vi "WILT Stave Status.vi"(0 "GUI Aisle 4":T3[](array[typedef]) {"Night Cycle Count" format="%04d"; "Day Cycle Count" format="%04d"}, 1 "Operation Type":enum16{"Write", "Read"}(ring), 2 "File Locations":T1[](array[typedef]), 5 "GUI Aisle 3":T3[](array[typedef]) {"Night Cycle Count" format="%04d"; "Day Cycle Count" format="%04d"}, 7 "GUI Aisle 2":T3[](array[typedef]) {"Night Cycle Count" format="%04d"; "Day Cycle Count" format="%04d"}, 9 "GUI Aisle 1 (SLAT)":T3[](array[typedef]) {"Night Cycle Count" format="%04d"; "Day Cycle Count" format="%04d"}, 11 "Error In":errorcluster, 12 "GUI Aisle 1A (SLAT)":T3[](array[typedef]) {"Night Cycle Count" format="%04d"; "Day Cycle Count" format="%04d"}) -> (4 "GUI Aisle 4 Out":T3[](array[typedef]) {"Night Cycle Count" format="%04d"; "Day Cycle Count" format="%04d"}, 6 "GUI Aisle 3 Out":T3[](array[typedef]) {"Night Cycle Count" format="%04d"; "Day Cycle Count" format="%04d"}, 8 "GUI Aisle 2 Out":T3[](array[typedef]) {"Night Cycle Count" format="%04d"; "Day Cycle Count" format="%04d"}, 10 "GUI Aisle 1 (SLAT) Out":T3[](array[typedef]) {"Night Cycle Count" format="%04d"; "Day Cycle Count" format="%04d"}, 14 "GUI Aisle 1A (SLAT) Out":T3[](array[typedef]) {"Night Cycle Count" format="%04d"; "Day Cycle Count" format="%04d"}, 15 "Error Out":errorcluster)   [LabVIEW 2016]
uses:
  Type Definitions/WILT Dryer.ctl
  Type Definitions/WILT Dryer Details.ctl
  Type Definitions/WILT Agilent Channel Definition.ctl
  Type Definitions/WILT DAQ Data.ctl
  Utility/Save File/File Setup (Public)/Type Definition/Save File DOE File Path Control.ctl
  Utility/Save File/File Setup (Public)/Type Definition/Save File DOE Data Save Filepaths.ctl
  <vilib>/Utility/file.llb/Write Delimited Spreadsheet (string).vi
  <vilib>/Utility/file.llb/Read Delimited Spreadsheet (string).vi
  Utility/Save File/File Setup.lvlib
panel:
  out "Info Table":string[][](array[string])
  # "Day"
  # "Night"
  # "Day"
  # "Night"
  # "Day"
  # "Night"
  # "Day"
  # "Night"
  # "Day"
  # "Night"
  # "Day"
  # "Night"
  # "Day"
  # "Night"
  # "Day"
  # "Night"
  # "Day"
  # "Night"
  # "Day"
  # "Night"
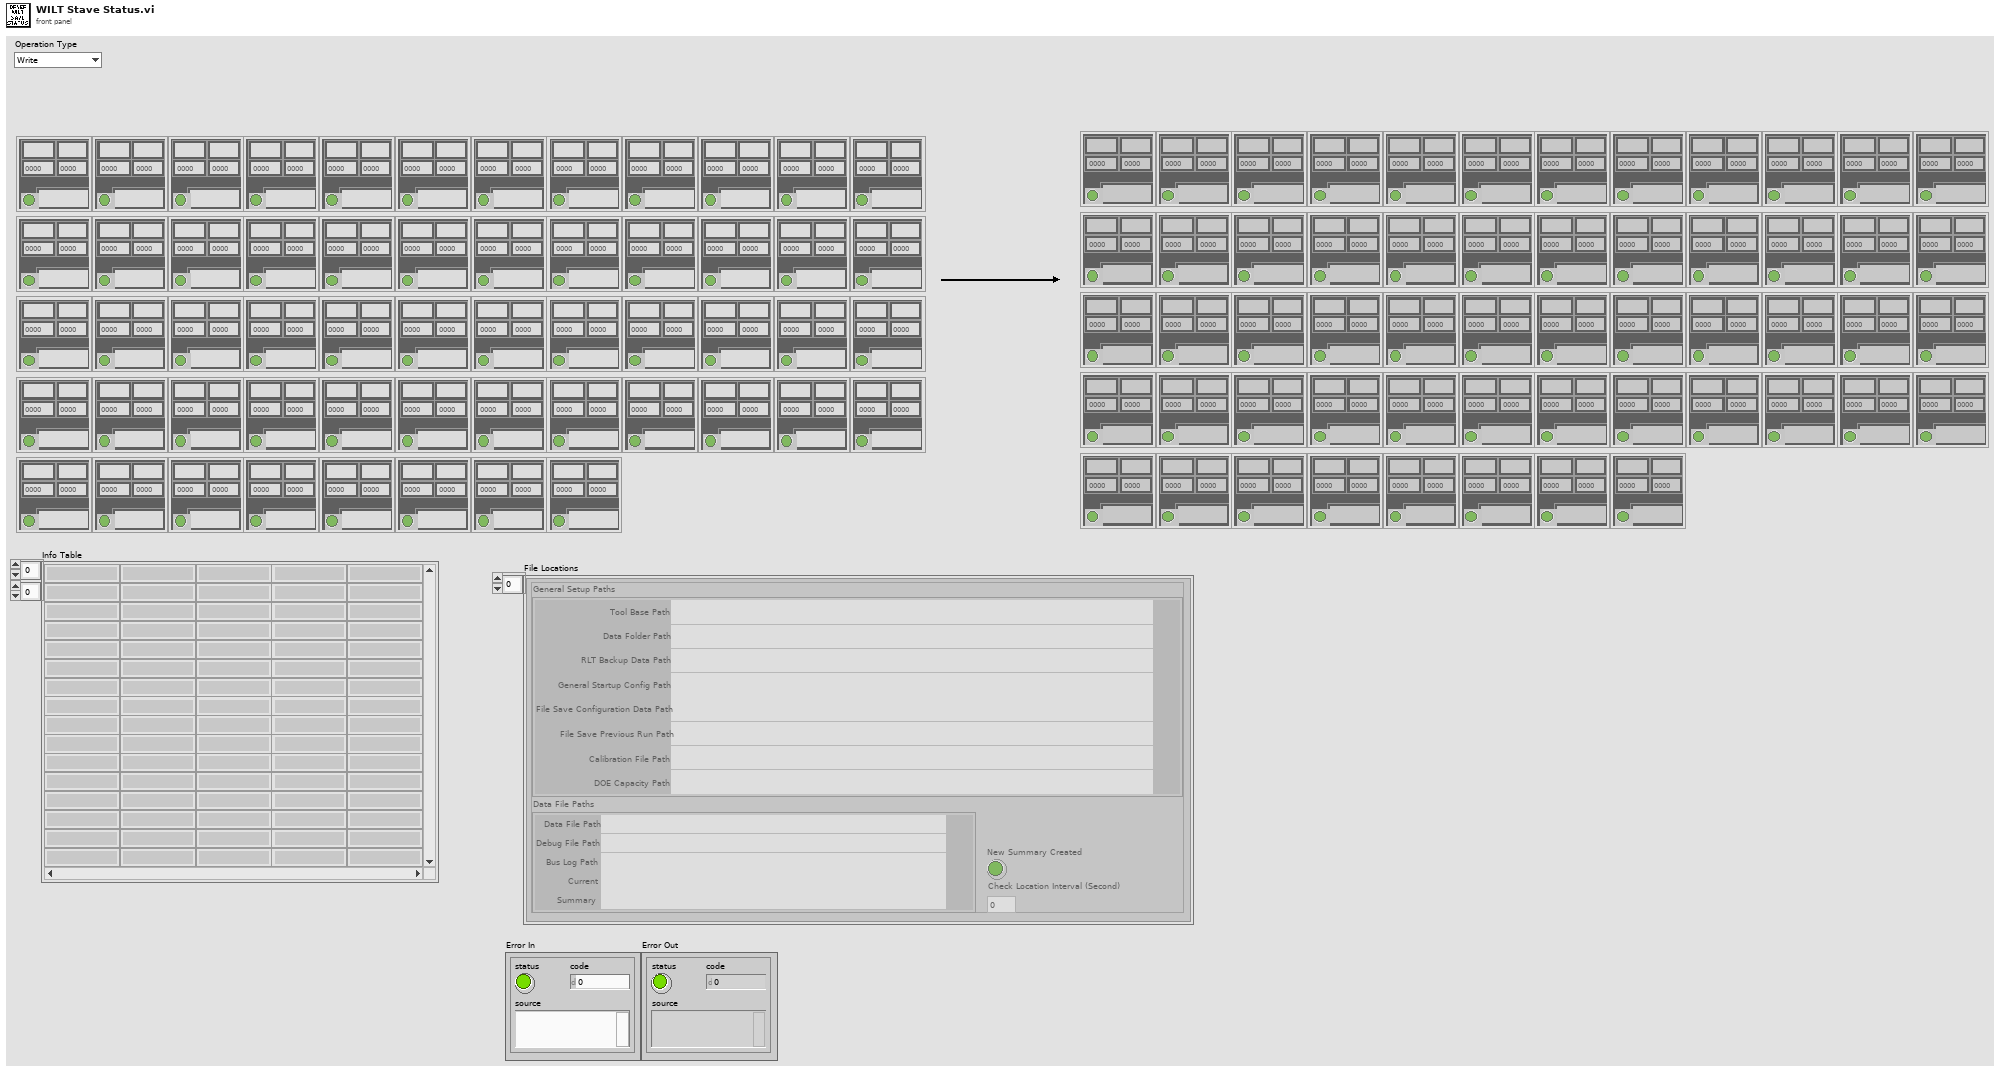
[diagram p1: front panel]
types:
  T1 = typedef "File Setup.lvlib/Save File DOE File Path Control.ctl" = cluster{"General Setup Paths":cluster{"Calibration File Path":path, "DOE Capacity Path":path, "Data Folder Path":path, "RLT Backup Data Path":path, "Tool Base Path":path, "General Startup Config Path":path, "File Save Previous Run Path":path, "File Save Configuration Data Path":path}, "Data File Paths":T2, "New Summary Created":bool, "Check Location Interval (Second)":i32}
  T2 = typedef "File Setup.lvlib/Save File DOE Data Save Filepaths.ctl" = cluster{"Data File Path":path, "Debug File Path":path, "Bus Log Path":path, "Current":path, "Summary":path}
  T3 = typedef "WILT Dryer.ctl" = cluster{"Lab ID":string, "Day Cycle Count":i32, "Station Label":string, "Dryer Details":T4, "Status Color":u32, "Invisible Button":bool, "Night Cycle Count":i32, "Station Index":i32, "Cycle Index":string, "Audit Alert":bool, "Agilent Channel Definition":T5, "DAQ Data":T6}
  T4 = typedef "WILT Dryer Details.ctl" = cluster{"Station":string, "Lab ID":string, "TR Number":string}
  T5 = typedef "WILT Agilent Channel Definition.ctl" = cluster{"Channel":string, "Station":string, "Label":string, "Agilent Station":string, "Data":dbl}
  T6 = typedef "WILT DAQ Data.ctl" = cluster{"L1 Current":dbl, "L2 Current":dbl, "Temperature  Deg F (TC)":dbl, "Volts":dbl, "Volts (208)":dbl, "SW (208)":dbl}
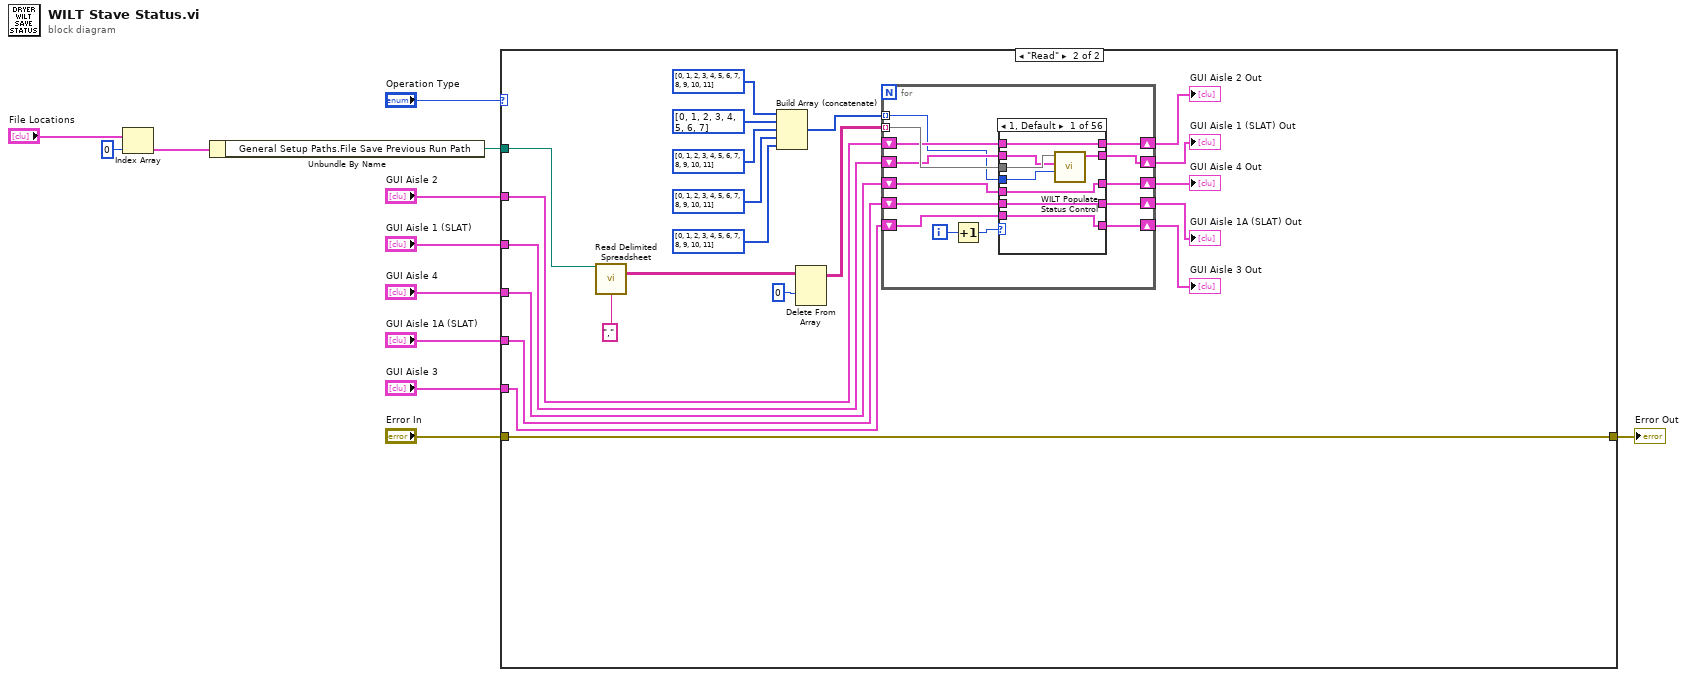
[diagram p0: block diagram]
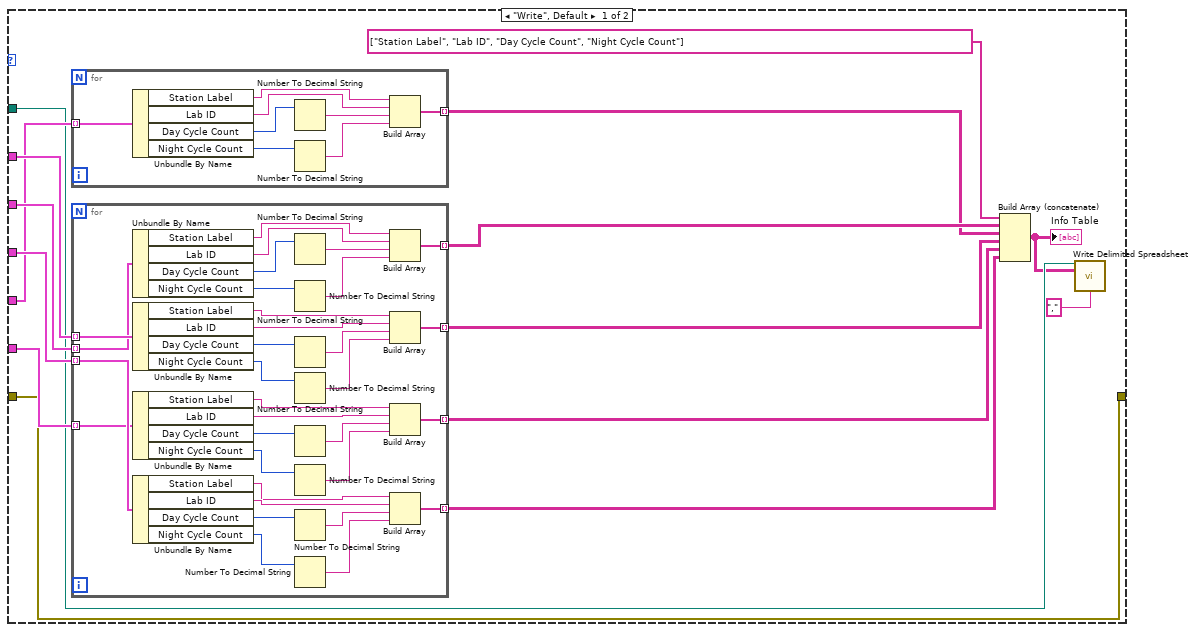
[diagram p2: hidden frame]
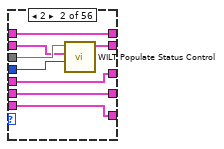
[diagram p3: hidden frame]
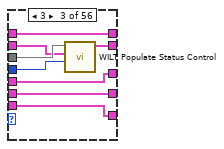
[diagram p4: hidden frame]
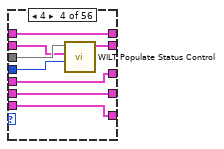
[diagram p5: hidden frame]
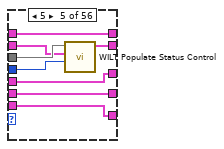
[diagram p6: hidden frame]
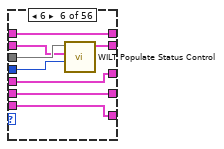
[diagram p7: hidden frame]
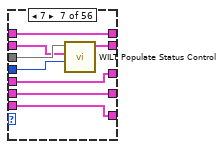
[diagram p8: hidden frame]
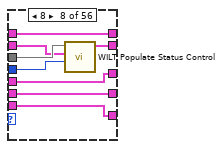
[diagram p9: hidden frame]
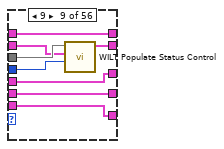
[diagram p10: hidden frame]
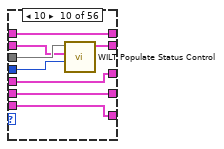
[diagram p11: hidden frame]
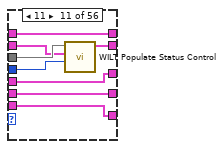
[diagram p12: hidden frame]
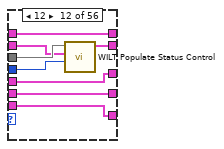
[diagram p13: hidden frame]
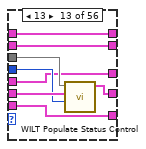
[diagram p14: hidden frame]
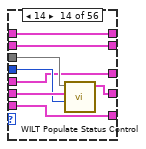
[diagram p15: hidden frame]
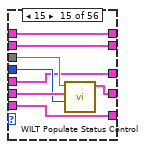
[diagram p16: hidden frame]
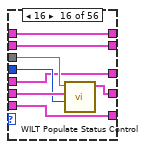
[diagram p17: hidden frame]
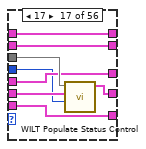
[diagram p18: hidden frame]
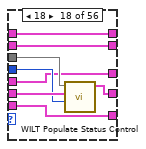
[diagram p19: hidden frame]
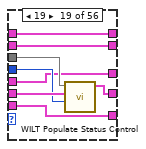
[diagram p20: hidden frame]
diagram:
  n1 = Index Array(array="File Locations", index=0) -> (element=w2:T1)
  n2 = Unbundle By Name(w2) -> ("General Setup Paths.File Save Previous Run Path"=w1:path)
  n3 = case shown="\"Read\"" "Operation Type" {
    tunnel: "GUI Aisle 4" -> [w27 w83]
    tunnel: "GUI Aisle 3" -> [w26 w84]
    tunnel: "GUI Aisle 2" -> [w25 w85]
    tunnel: "GUI Aisle 1 (SLAT)" -> [w24 w86]
    tunnel: "GUI Aisle 1A (SLAT)" -> [w23 w79]
    tunnel: w1 -> [w17 w88]
    tunnel: "Error In" -> [w15 w89]
    tunnel: [w15 w89] -> w5
    frame "Write", Default {
      n4 = for {
        tunnel: w23 -> [w28] mode=indexing
        tunnel: [w29] -> w21 mode=indexing
        n5 = Unbundle By Name(w28) -> ("Station Label"=w35:string, "Lab ID"=w34:string, "Day Cycle Count"=w33:i32, "Night Cycle Count"=w31:i32)
        n6 = Number To Decimal String(number=w33) -> (decimal integer string=w32:string)  [unwired: 1 in]
        n7 = Number To Decimal String(number=w31) -> (decimal integer string=w30:string)  [unwired: 1 in]
        n8 = Build Array(w35, w34, w32, w30) -> (w29:string[])
      }
      n9 = for {
        tunnel: w27 -> [w67] mode=indexing
        tunnel: w26 -> [w66] mode=indexing
        tunnel: w25 -> [w65] mode=indexing
        tunnel: w24 -> [w64] mode=indexing
        tunnel: [w43] -> w18 mode=indexing
        tunnel: [w42] -> w19 mode=indexing
        tunnel: [w41] -> w20 mode=indexing
        tunnel: [w40] -> w22 mode=indexing
        n10 = Unbundle By Name(w64) -> ("Station Label"=w36:string, "Lab ID"=w46:string, "Day Cycle Count"=w57:i32, "Night Cycle Count"=w56:i32)
        n11 = Unbundle By Name(w65) -> ("Station Label"=w37:string, "Lab ID"=w49:string, "Day Cycle Count"=w59:i32, "Night Cycle Count"=w58:i32)
        n12 = Unbundle By Name(w66) -> ("Station Label"=w38:string, "Lab ID"=w52:string, "Day Cycle Count"=w61:i32, "Night Cycle Count"=w60:i32)
        n13 = Unbundle By Name(w67) -> ("Station Label"=w39:string, "Lab ID"=w55:string, "Day Cycle Count"=w63:i32, "Night Cycle Count"=w62:i32)
        n14 = Number To Decimal String(number=w57) -> (decimal integer string=w45:string)  [unwired: 1 in]
        n15 = Number To Decimal String(number=w56) -> (decimal integer string=w44:string)  [unwired: 1 in]
        n16 = Number To Decimal String(number=w59) -> (decimal integer string=w48:string)  [unwired: 1 in]
        n17 = Number To Decimal String(number=w58) -> (decimal integer string=w47:string)  [unwired: 1 in]
        n18 = Number To Decimal String(number=w61) -> (decimal integer string=w51:string)  [unwired: 1 in]
        n19 = Number To Decimal String(number=w60) -> (decimal integer string=w50:string)  [unwired: 1 in]
        n20 = Number To Decimal String(number=w63) -> (decimal integer string=w54:string)  [unwired: 1 in]
        n21 = Number To Decimal String(number=w62) -> (decimal integer string=w53:string)  [unwired: 1 in]
        n22 = Build Array(w36, w46, w45, w44) -> (w40:string[])
        n23 = Build Array(w37, w49, w48, w47) -> (w41:string[])
        n24 = Build Array(w38, w52, w51, w50) -> (w42:string[])
        n25 = Build Array(w39, w55, w54, w53) -> (w43:string[])
      }
      n26 = Build Array (concatenate)(string[] ["Station Label", "Lab ID", "Day Cycle Count", "Night Cycle Count"], w22, w21, w20, w19, w18) -> (w13:string[][])
      "Info Table" <- w13
      n27 = call-poly <vilib>:"Write Delimited Spreadsheet.vi"("file path (dialog if empty)"=w17, "2D data"=w13, "delimiter (\\t)"="," ("delimiter (\\t)")) -> ()  [unwired: 11 in, 2 out]
    }
    frame "Read" {
      n28 = call-poly <vilib>:"Read Delimited Spreadsheet.vi"("file path (dialog if empty)"=w88, "delimiter (\\t)"="," ("delimiter (\\t)")) -> ("all rows"=w68:string[][])  [unwired: 8 in, 5 out]
      n29 = Build Array (concatenate)(i32[] [0, 1, 2, 3, 4, 5, 6, 7, 8, 9, 10, 11], i32[] [0, 1, 2, 3, 4, 5, 6, 7], i32[] [0, 1, 2, 3, 4, 5, 6, 7, 8, 9, 10, 11], i32[] [0, 1, 2, 3, 4, 5, 6, 7, 8, 9, 10, 11], i32[] [0, 1, 2, 3, 4, 5, 6, 7, 8, 9, 10, 11]) -> (w69:i32[])
      n30 = Delete From Array(array=w68, index (row)=0) -> (array with subset deleted=w81:string[][])  [unwired: 2 in, 1 out]
      n31 = for {
        tunnel: w81 -> [w102] mode=indexing
        shift-right: [w99] -> w80
        shift-left: w86 -> [w101]
        shift-right: [w97] -> w78
        shift-left: w79 -> [w98]
        shift-right: [w95] -> w77
        shift-left: w85 -> [w96]
        shift-right: [w93] -> w76
        shift-left: w84 -> [w94]
        shift-right: [w91] -> w75
        shift-left: w83 -> [w92]
        tunnel: w69 -> [w90] mode=indexing
        i -> [w100]
        n32 = Increment(x=w100) -> (x+1=w103:i32)
        n33 = case shown="1, Default" w103 {
          tunnel: w102 -> [w111 w119 w127 w135 w143 w151 w159 w167 w175 w183 w191 w199 w207 w215 w223 w231 w239 w247 w255 w263 w271 w279 w287 w295 w303 w311 w318 w327 w335 w343 w351 w359 w367 w375 w382 w391 w399 w407 w415 w423 w430 w439 w446 w455 w462 w471 w478 w487 w494 w502 w511 w519 w527 w535 w543 w551]
          tunnel: w101 -> [w110 w118 w126 w134 w142 w149 w158 w166 w173 w182 w189 w198 w203 w211 w219 w227 w236 w242 w251 w259 w267 w274 w282 w291 w298 w306 w314 w322 w331 w339 w346 w354 w362 w370 w378 w386 w394 w402 w410 w418 w426 w434 w442 w450 w458 w466 w474 w482 w490 w498 w506 w514 w522 w530 w538 w546]
          tunnel: w90 -> [w109 w116 w124 w132 w140 w148 w156 w164 w172 w180 w188 w197 w205 w213 w221 w228 w232 w244 w252 w260 w266 w276 w284 w292 w301 w308 w316 w324 w332 w340 w349 w357 w365 w372 w381 w389 w396 w404 w412 w421 w431 w437 w445 w453 w461 w469 w479 w484 w493 w501 w510 w517 w526 w533 w541 w549]
          tunnel: [w108 w117 w125 w133 w141 w150 w157 w165 w174 w181 w190 w196 w203 w211 w219 w227 w236 w242 w251 w259 w267 w274 w282 w291 w298 w306 w314 w322 w331 w339 w346 w354 w362 w370 w378 w386 w394 w402 w410 w418 w426 w434 w442 w450 w458 w466 w474 w482 w490 w498 w506 w514 w522 w530 w538 w546] -> w99
          tunnel: w98 -> [w105 w113 w121 w129 w137 w145 w153 w161 w169 w177 w185 w193 w206 w214 w222 w230 w238 w246 w253 w262 w268 w275 w283 w289 w299 w307 w315 w323 w329 w337 w347 w355 w360 w368 w377 w384 w392 w400 w408 w416 w424 w432 w440 w448 w457 w465 w473 w481 w489 w497 w505 w513 w521 w529 w537 w545]
          tunnel: [w105 w113 w121 w129 w137 w145 w153 w161 w169 w177 w185 w193 w204 w212 w220 w229 w237 w245 w254 w261 w268 w275 w283 w289 w299 w307 w315 w323 w329 w337 w347 w355 w360 w368 w377 w384 w392 w400 w408 w416 w424 w432 w440 w448 w457 w465 w473 w481 w489 w497 w505 w513 w521 w529 w537 w545] -> w97
          tunnel: w96 -> [w107 w115 w123 w131 w139 w147 w155 w163 w171 w179 w187 w195 w202 w210 w218 w226 w235 w243 w250 w258 w270 w278 w286 w294 w302 w309 w319 w326 w333 w341 w350 w358 w363 w371 w379 w387 w395 w403 w411 w419 w427 w435 w443 w451 w459 w467 w475 w483 w491 w499 w507 w515 w523 w531 w539 w547]
          tunnel: [w107 w115 w123 w131 w139 w147 w155 w163 w171 w179 w187 w195 w202 w210 w218 w226 w235 w243 w250 w258 w269 w277 w285 w293 w300 w310 w317 w325 w334 w342 w348 w356 w363 w371 w379 w387 w395 w403 w411 w419 w427 w435 w443 w451 w459 w467 w475 w483 w491 w499 w507 w515 w523 w531 w539 w547] -> w95
          tunnel: w94 -> [w104 w112 w120 w128 w136 w144 w152 w160 w168 w176 w184 w192 w200 w208 w216 w224 w233 w240 w248 w256 w264 w272 w280 w288 w296 w304 w312 w320 w328 w336 w344 w352 w366 w374 w383 w390 w398 w406 w414 w422 w429 w438 w447 w454 w456 w464 w472 w480 w488 w496 w504 w512 w520 w528 w536 w544]
          tunnel: [w104 w112 w120 w128 w136 w144 w152 w160 w168 w176 w184 w192 w200 w208 w216 w224 w233 w240 w248 w256 w264 w272 w280 w288 w296 w304 w312 w320 w328 w336 w344 w352 w364 w373 w380 w388 w397 w405 w413 w420 w428 w436 w444 w452 w456 w464 w472 w480 w488 w496 w504 w512 w520 w528 w536 w544] -> w93
          tunnel: w92 -> [w106 w114 w122 w130 w138 w146 w154 w162 w170 w178 w186 w194 w201 w209 w217 w225 w234 w241 w249 w257 w265 w273 w281 w290 w297 w305 w313 w321 w330 w338 w345 w353 w361 w369 w376 w385 w393 w401 w409 w417 w425 w433 w441 w449 w463 w470 w477 w486 w495 w503 w509 w518 w525 w534 w542 w550]
          tunnel: [w106 w114 w122 w130 w138 w146 w154 w162 w170 w178 w186 w194 w201 w209 w217 w225 w234 w241 w249 w257 w265 w273 w281 w290 w297 w305 w313 w321 w330 w338 w345 w353 w361 w369 w376 w385 w393 w401 w409 w417 w425 w433 w441 w449 w460 w468 w476 w485 w492 w500 w508 w516 w524 w532 w540 w548] -> w91
          frame 1, Default {
            n34 = call "WILT Populate Status Control.vi"("Index"=w109, "GUI Aisle 1 (SLAT) in"=w110, "Raw Data From File"=w111) -> ("GUI Aisle 1 (SLAT) out"=w108:T3[])  [unwired: 8 in]
          }
          frame 2 {
            n35 = call "WILT Populate Status Control.vi"("Index"=w116, "GUI Aisle 1 (SLAT) in"=w118, "Raw Data From File"=w119) -> ("GUI Aisle 1 (SLAT) out"=w117:T3[])  [unwired: 8 in]
          }
          frame 3 {
            n36 = call "WILT Populate Status Control.vi"("Index"=w124, "GUI Aisle 1 (SLAT) in"=w126, "Raw Data From File"=w127) -> ("GUI Aisle 1 (SLAT) out"=w125:T3[])  [unwired: 8 in]
          }
          frame 4 {
            n37 = call "WILT Populate Status Control.vi"("Index"=w132, "GUI Aisle 1 (SLAT) in"=w134, "Raw Data From File"=w135) -> ("GUI Aisle 1 (SLAT) out"=w133:T3[])  [unwired: 8 in]
          }
          frame 5 {
            n38 = call "WILT Populate Status Control.vi"("Index"=w140, "GUI Aisle 1 (SLAT) in"=w142, "Raw Data From File"=w143) -> ("GUI Aisle 1 (SLAT) out"=w141:T3[])  [unwired: 8 in]
          }
          frame 6 {
            n39 = call "WILT Populate Status Control.vi"("Index"=w148, "GUI Aisle 1 (SLAT) in"=w149, "Raw Data From File"=w151) -> ("GUI Aisle 1 (SLAT) out"=w150:T3[])  [unwired: 8 in]
          }
          frame 7 {
            n40 = call "WILT Populate Status Control.vi"("Index"=w156, "GUI Aisle 1 (SLAT) in"=w158, "Raw Data From File"=w159) -> ("GUI Aisle 1 (SLAT) out"=w157:T3[])  [unwired: 8 in]
          }
          frame 8 {
            n41 = call "WILT Populate Status Control.vi"("Index"=w164, "GUI Aisle 1 (SLAT) in"=w166, "Raw Data From File"=w167) -> ("GUI Aisle 1 (SLAT) out"=w165:T3[])  [unwired: 8 in]
          }
          frame 9 {
            n42 = call "WILT Populate Status Control.vi"("Index"=w172, "GUI Aisle 1 (SLAT) in"=w173, "Raw Data From File"=w175) -> ("GUI Aisle 1 (SLAT) out"=w174:T3[])  [unwired: 8 in]
          }
          frame 10 {
            n43 = call "WILT Populate Status Control.vi"("Index"=w180, "GUI Aisle 1 (SLAT) in"=w182, "Raw Data From File"=w183) -> ("GUI Aisle 1 (SLAT) out"=w181:T3[])  [unwired: 8 in]
          }
          frame 11 {
            n44 = call "WILT Populate Status Control.vi"("Index"=w188, "GUI Aisle 1 (SLAT) in"=w189, "Raw Data From File"=w191) -> ("GUI Aisle 1 (SLAT) out"=w190:T3[])  [unwired: 8 in]
          }
          frame 12 {
            n45 = call "WILT Populate Status Control.vi"("Index"=w197, "GUI Aisle 1 (SLAT) in"=w198, "Raw Data From File"=w199) -> ("GUI Aisle 1 (SLAT) out"=w196:T3[])  [unwired: 8 in]
          }
          frame 13 {
            n46 = call "WILT Populate Status Control.vi"("Index"=w205, "GUI Aisle 1 (SLAT) in"=w206, "Raw Data From File"=w207) -> ("GUI Aisle 1 (SLAT) out"=w204:T3[])  [unwired: 8 in]
          }
          frame 14 {
            n47 = call "WILT Populate Status Control.vi"("Index"=w213, "GUI Aisle 1 (SLAT) in"=w214, "Raw Data From File"=w215) -> ("GUI Aisle 1 (SLAT) out"=w212:T3[])  [unwired: 8 in]
          }
          frame 15 {
            n48 = call "WILT Populate Status Control.vi"("Index"=w221, "GUI Aisle 1 (SLAT) in"=w222, "Raw Data From File"=w223) -> ("GUI Aisle 1 (SLAT) out"=w220:T3[])  [unwired: 8 in]
          }
          frame 16 {
            n49 = call "WILT Populate Status Control.vi"("Index"=w228, "GUI Aisle 1 (SLAT) in"=w230, "Raw Data From File"=w231) -> ("GUI Aisle 1 (SLAT) out"=w229:T3[])  [unwired: 8 in]
          }
          frame 17 {
            n50 = call "WILT Populate Status Control.vi"("Index"=w232, "GUI Aisle 1 (SLAT) in"=w238, "Raw Data From File"=w239) -> ("GUI Aisle 1 (SLAT) out"=w237:T3[])  [unwired: 8 in]
          }
          frame 18 {
            n51 = call "WILT Populate Status Control.vi"("Index"=w244, "GUI Aisle 1 (SLAT) in"=w246, "Raw Data From File"=w247) -> ("GUI Aisle 1 (SLAT) out"=w245:T3[])  [unwired: 8 in]
          }
          frame 19 {
            n52 = call "WILT Populate Status Control.vi"("Index"=w252, "GUI Aisle 1 (SLAT) in"=w253, "Raw Data From File"=w255) -> ("GUI Aisle 1 (SLAT) out"=w254:T3[])  [unwired: 8 in]
          }
          frame 20 {
            n53 = call "WILT Populate Status Control.vi"("Index"=w260, "GUI Aisle 1 (SLAT) in"=w262, "Raw Data From File"=w263) -> ("GUI Aisle 1 (SLAT) out"=w261:T3[])  [unwired: 8 in]
          }
          frame 21 {
            n54 = call "WILT Populate Status Control.vi"("Index"=w266, "GUI Aisle 1 (SLAT) in"=w270, "Raw Data From File"=w271) -> ("GUI Aisle 1 (SLAT) out"=w269:T3[])  [unwired: 8 in]
          }
          frame 22 {
            n55 = call "WILT Populate Status Control.vi"("Index"=w276, "GUI Aisle 1 (SLAT) in"=w278, "Raw Data From File"=w279) -> ("GUI Aisle 1 (SLAT) out"=w277:T3[])  [unwired: 8 in]
          }
          frame 23 {
            n56 = call "WILT Populate Status Control.vi"("Index"=w284, "GUI Aisle 1 (SLAT) in"=w286, "Raw Data From File"=w287) -> ("GUI Aisle 1 (SLAT) out"=w285:T3[])  [unwired: 8 in]
          }
          frame 24 {
            n57 = call "WILT Populate Status Control.vi"("Index"=w292, "GUI Aisle 1 (SLAT) in"=w294, "Raw Data From File"=w295) -> ("GUI Aisle 1 (SLAT) out"=w293:T3[])  [unwired: 8 in]
          }
          frame 25 {
            n58 = call "WILT Populate Status Control.vi"("Index"=w301, "GUI Aisle 1 (SLAT) in"=w302, "Raw Data From File"=w303) -> ("GUI Aisle 1 (SLAT) out"=w300:T3[])  [unwired: 8 in]
          }
          frame 26 {
            n59 = call "WILT Populate Status Control.vi"("Index"=w308, "GUI Aisle 1 (SLAT) in"=w309, "Raw Data From File"=w311) -> ("GUI Aisle 1 (SLAT) out"=w310:T3[])  [unwired: 8 in]
          }
          frame 27 {
            n60 = call "WILT Populate Status Control.vi"("Index"=w316, "GUI Aisle 1 (SLAT) in"=w319, "Raw Data From File"=w318) -> ("GUI Aisle 1 (SLAT) out"=w317:T3[])  [unwired: 8 in]
          }
          frame 28 {
            n61 = call "WILT Populate Status Control.vi"("Index"=w324, "GUI Aisle 1 (SLAT) in"=w326, "Raw Data From File"=w327) -> ("GUI Aisle 1 (SLAT) out"=w325:T3[])  [unwired: 8 in]
          }
          frame 29 {
            n62 = call "WILT Populate Status Control.vi"("Index"=w332, "GUI Aisle 1 (SLAT) in"=w333, "Raw Data From File"=w335) -> ("GUI Aisle 1 (SLAT) out"=w334:T3[])  [unwired: 8 in]
          }
          frame 30 {
            n63 = call "WILT Populate Status Control.vi"("Index"=w340, "GUI Aisle 1 (SLAT) in"=w341, "Raw Data From File"=w343) -> ("GUI Aisle 1 (SLAT) out"=w342:T3[])  [unwired: 8 in]
          }
          frame 31 {
            n64 = call "WILT Populate Status Control.vi"("Index"=w349, "GUI Aisle 1 (SLAT) in"=w350, "Raw Data From File"=w351) -> ("GUI Aisle 1 (SLAT) out"=w348:T3[])  [unwired: 8 in]
          }
          frame 32 {
            n65 = call "WILT Populate Status Control.vi"("Index"=w357, "GUI Aisle 1 (SLAT) in"=w358, "Raw Data From File"=w359) -> ("GUI Aisle 1 (SLAT) out"=w356:T3[])  [unwired: 8 in]
          }
          frame 33 {
            n66 = call "WILT Populate Status Control.vi"("Index"=w365, "GUI Aisle 1 (SLAT) in"=w366, "Raw Data From File"=w367) -> ("GUI Aisle 1 (SLAT) out"=w364:T3[])  [unwired: 8 in]
          }
          frame 34 {
            n67 = call "WILT Populate Status Control.vi"("Index"=w372, "GUI Aisle 1 (SLAT) in"=w374, "Raw Data From File"=w375) -> ("GUI Aisle 1 (SLAT) out"=w373:T3[])  [unwired: 8 in]
          }
          frame 35 {
            n68 = call "WILT Populate Status Control.vi"("Index"=w381, "GUI Aisle 1 (SLAT) in"=w383, "Raw Data From File"=w382) -> ("GUI Aisle 1 (SLAT) out"=w380:T3[])  [unwired: 8 in]
          }
          frame 36 {
            n69 = call "WILT Populate Status Control.vi"("Index"=w389, "GUI Aisle 1 (SLAT) in"=w390, "Raw Data From File"=w391) -> ("GUI Aisle 1 (SLAT) out"=w388:T3[])  [unwired: 8 in]
          }
          frame 37 {
            n70 = call "WILT Populate Status Control.vi"("Index"=w396, "GUI Aisle 1 (SLAT) in"=w398, "Raw Data From File"=w399) -> ("GUI Aisle 1 (SLAT) out"=w397:T3[])  [unwired: 8 in]
          }
          frame 38 {
            n71 = call "WILT Populate Status Control.vi"("Index"=w404, "GUI Aisle 1 (SLAT) in"=w406, "Raw Data From File"=w407) -> ("GUI Aisle 1 (SLAT) out"=w405:T3[])  [unwired: 8 in]
          }
          frame 39 {
            n72 = call "WILT Populate Status Control.vi"("Index"=w412, "GUI Aisle 1 (SLAT) in"=w414, "Raw Data From File"=w415) -> ("GUI Aisle 1 (SLAT) out"=w413:T3[])  [unwired: 8 in]
          }
          frame 40 {
            n73 = call "WILT Populate Status Control.vi"("Index"=w421, "GUI Aisle 1 (SLAT) in"=w422, "Raw Data From File"=w423) -> ("GUI Aisle 1 (SLAT) out"=w420:T3[])  [unwired: 8 in]
          }
          frame 41 {
            n74 = call "WILT Populate Status Control.vi"("Index"=w431, "GUI Aisle 1 (SLAT) in"=w429, "Raw Data From File"=w430) -> ("GUI Aisle 1 (SLAT) out"=w428:T3[])  [unwired: 8 in]
          }
          frame 42 {
            n75 = call "WILT Populate Status Control.vi"("Index"=w437, "GUI Aisle 1 (SLAT) in"=w438, "Raw Data From File"=w439) -> ("GUI Aisle 1 (SLAT) out"=w436:T3[])  [unwired: 8 in]
          }
          frame 43 {
            n76 = call "WILT Populate Status Control.vi"("Index"=w445, "GUI Aisle 1 (SLAT) in"=w447, "Raw Data From File"=w446) -> ("GUI Aisle 1 (SLAT) out"=w444:T3[])  [unwired: 8 in]
          }
          frame 44 {
            n77 = call "WILT Populate Status Control.vi"("Index"=w453, "GUI Aisle 1 (SLAT) in"=w454, "Raw Data From File"=w455) -> ("GUI Aisle 1 (SLAT) out"=w452:T3[])  [unwired: 8 in]
          }
          frame 45 {
            n78 = call "WILT Populate Status Control.vi"("Index"=w461, "GUI Aisle 1 (SLAT) in"=w463, "Raw Data From File"=w462) -> ("GUI Aisle 1 (SLAT) out"=w460:T3[])  [unwired: 8 in]
          }
          frame 46 {
            n79 = call "WILT Populate Status Control.vi"("Index"=w469, "GUI Aisle 1 (SLAT) in"=w470, "Raw Data From File"=w471) -> ("GUI Aisle 1 (SLAT) out"=w468:T3[])  [unwired: 8 in]
          }
          frame 47 {
            n80 = call "WILT Populate Status Control.vi"("Index"=w479, "GUI Aisle 1 (SLAT) in"=w477, "Raw Data From File"=w478) -> ("GUI Aisle 1 (SLAT) out"=w476:T3[])  [unwired: 8 in]
          }
          frame 48 {
            n81 = call "WILT Populate Status Control.vi"("Index"=w484, "GUI Aisle 1 (SLAT) in"=w486, "Raw Data From File"=w487) -> ("GUI Aisle 1 (SLAT) out"=w485:T3[])  [unwired: 8 in]
          }
          frame 49 {
            n82 = call "WILT Populate Status Control.vi"("Index"=w493, "GUI Aisle 1 (SLAT) in"=w495, "Raw Data From File"=w494) -> ("GUI Aisle 1 (SLAT) out"=w492:T3[])  [unwired: 8 in]
          }
          frame 50 {
            n83 = call "WILT Populate Status Control.vi"("Index"=w501, "GUI Aisle 1 (SLAT) in"=w503, "Raw Data From File"=w502) -> ("GUI Aisle 1 (SLAT) out"=w500:T3[])  [unwired: 8 in]
          }
          frame 51 {
            n84 = call "WILT Populate Status Control.vi"("Index"=w510, "GUI Aisle 1 (SLAT) in"=w509, "Raw Data From File"=w511) -> ("GUI Aisle 1 (SLAT) out"=w508:T3[])  [unwired: 8 in]
          }
          frame 52 {
            n85 = call "WILT Populate Status Control.vi"("Index"=w517, "GUI Aisle 1 (SLAT) in"=w518, "Raw Data From File"=w519) -> ("GUI Aisle 1 (SLAT) out"=w516:T3[])  [unwired: 8 in]
          }
          frame 53 {
            n86 = call "WILT Populate Status Control.vi"("Index"=w526, "GUI Aisle 1 (SLAT) in"=w525, "Raw Data From File"=w527) -> ("GUI Aisle 1 (SLAT) out"=w524:T3[])  [unwired: 8 in]
          }
          frame 54 {
            n87 = call "WILT Populate Status Control.vi"("Index"=w533, "GUI Aisle 1 (SLAT) in"=w534, "Raw Data From File"=w535) -> ("GUI Aisle 1 (SLAT) out"=w532:T3[])  [unwired: 8 in]
          }
          frame 55 {
            n88 = call "WILT Populate Status Control.vi"("Index"=w541, "GUI Aisle 1 (SLAT) in"=w542, "Raw Data From File"=w543) -> ("GUI Aisle 1 (SLAT) out"=w540:T3[])  [unwired: 8 in]
          }
          frame 56 {
            n89 = call "WILT Populate Status Control.vi"("Index"=w549, "GUI Aisle 1 (SLAT) in"=w550, "Raw Data From File"=w551) -> ("GUI Aisle 1 (SLAT) out"=w548:T3[])  [unwired: 8 in]
          }
        }
      }
      "GUI Aisle 1A (SLAT) Out" <- w78
      "GUI Aisle 1 (SLAT) Out" <- w80
      "GUI Aisle 2 Out" <- w77
      "GUI Aisle 3 Out" <- w76
      "GUI Aisle 4 Out" <- w75
    }
  }
  "Error Out" <- w5
